vi "IdentityCheck.vi"(8 "error in (no error)":errorcluster, 11 "Class 4 in":refnum<class "Class 4.lvclass">) -> (0 "error out":errorcluster, 3 "Class 4 out":refnum<class "Class 4.lvclass">)   [LabVIEW 2013, in "Class 4.lvclass"]
doc: "An das Gerät wird eine Nachricht geschickt, in der Regel der Befehl idn?. Anhand der Antwort kann erkannt werden ob das erwartete Gerät angeschlossen ist."
uses:
  Class 4.lvclass
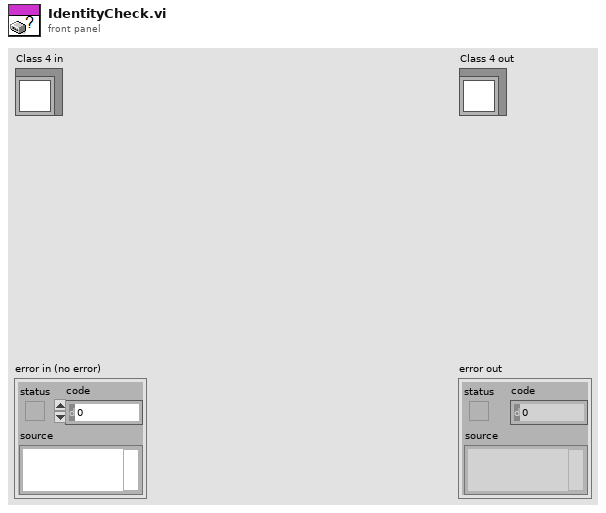
[diagram p1: front panel]
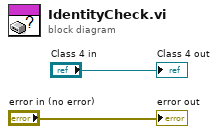
[diagram p0: block diagram]
diagram:
  "error out" <- "error in (no error)"
  "Class 4 out" <- "Class 4 in"
